vi "IIR Filter for N Chan.vi"(4 "optional IIR filter specifications":T3={"Lower PB"=100.0, "Upper PB"=0.0, "Lower SB"=200.0, "Upper SB"=0.0, "PB Gain"=0.0, "SB Gain"=-60.0, "Scale"=TRUE} {"PB Gain" format="%0.2f"; "SB Gain" format="%0.2f"; "Lower SB" format="%0.2p"; "Upper SB" format="%0.2f"; "Lower PB" format="%0.2p"; "Upper PB" format="%0.2f"}, 6 "IIR filter specifications":T4={"Topology"=enum."Butterworth", "Type"=enum."Lowpass", "Order"=1, "Lower Fc"=100.0, "Upper Fc"=200.0, "PB Ripple"=1.0, "SB Attenuation"=60.0} {"PB Ripple" format="%0.2f"; "SB Attenuation" format="%0.2f"; "Lower Fc" format="%0.2p"; "Upper Fc" format="%0.2p"}, 7 "reset filters":bool, 8 "error in (no error)":errorcluster, 10 "filter structure option":T1=10 items=["IIR 2nd Order"=0, "IIR 4th Order"=1, "Auto Select"=10], 11 "signal(s) in":waveform(dbl)[](array[waveform])) -> (0 "error out":errorcluster, 2 "filter information":T2 {"phase H(w)"."df" format="%.2p"; "phase H(w)"."f0" format="%.2p"; "phase H(w)"."Phase H(w)" format="%.2p"; "magnitude H(w)"."df" format="%.2p"; "magnitude H(w)"."f0" format="%.2p"; "magnitude H(w)"."Mag H(w)" format="%.2p"}, 3 "signal(s) out":waveform(dbl)[](array[waveform]))   [LabVIEW 2020, in "NI_MAPro.lvlib"]
doc: "Filters signals in either single or multiple waveforms. If you are filtering multiple waveforms, the VI maintains separate filter states for each waveform. The data types you wire to the <B>signal in</B> and <B>IIR filter specifications</B> inputs determine the polymorphic instance to use."
uses:
  NI_MAPro.lvlib
  Filter Structure Type.ctl
  NI_MABase.lvlib
  NI_AALBase.lvlib
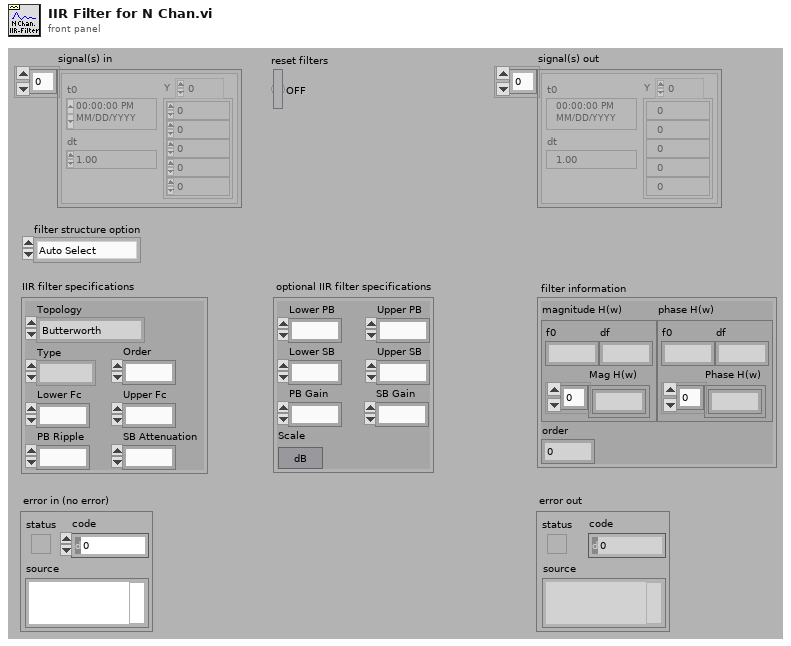
[diagram p1: front panel]
types:
  T1 = typedef "NI_AALBase.lvlib/Filter Structure Type.ctl" = u16
  T2 = cluster{"magnitude H(w)":cluster{"f0":dbl, "df":dbl, "Mag H(w)":dbl[]}, "phase H(w)":cluster{"f0":dbl, "df":dbl, "Phase H(w)":dbl[]}, "order":i32}
  T3 = cluster{"Lower PB":dbl, "Upper PB":dbl, "Lower SB":dbl, "Upper SB":dbl, "PB Gain":dbl, "SB Gain":dbl, "Scale":bool}
  T4 = cluster{"Topology":enum16{"Off", "Butterworth", "Chebyshev", "Inverse Chebyshev", "Elliptic", "Bessel"}, "Type":enum16{"Lowpass", "Highpass", "Bandpass", "Bandstop"}, "Order":i32, "Lower Fc":dbl, "Upper Fc":dbl, "PB Ripple":dbl, "SB Attenuation":dbl}
  T5 = cluster{"filter structure":enum32{"IIR 2nd Order", "IIR 4th Order"}, "Reverse Coefficients":dbl[], "Forward Coefficients":dbl[]}
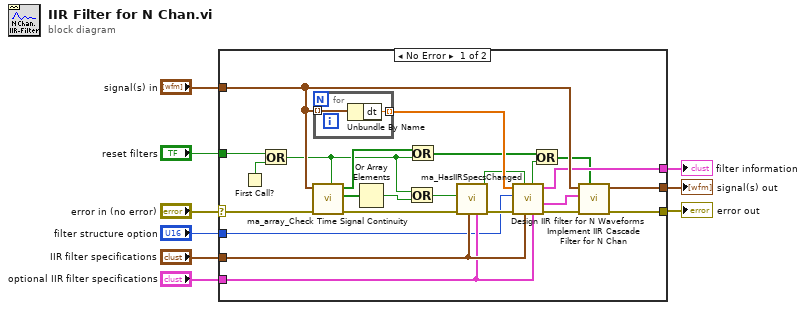
[diagram p0: block diagram]
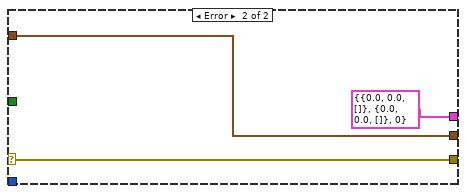
[diagram p2: hidden frame]
diagram:
  n1 = case shown="No Error" "error in (no error)" {
    selector: "error in (no error)" -> [w30 w37]
    tunnel: "signal(s) in" -> [w32 w38]
    tunnel: [w33 w37] -> w8
    tunnel: [w31 w38] -> w7
    tunnel: [w29 T2 {"magnitude H(w)"={"f0"=0.0, "df"=0.0, "Mag H(w)"=[]}, "phase H(w)"={"f0"=0.0, "df"=0.0, "Phase H(w)"=[]}, "order"=0} ("Filter Information")] -> w5
    tunnel: "reset filters" -> [w13 _]
    tunnel: "IIR filter specifications" -> [w12 _]
    tunnel: "optional IIR filter specifications" -> [w11 _]
    tunnel: "filter structure option" -> [w10 _]
    frame No Error {
      n2 = First Call?() -> (First Call?: T/F=w15:bool)
      n3 = Or(x=w13, y=w15) -> (x .or. y?=w14:bool)
      n4 = call "ma_array_Check Time Signal Continuity.vi"("Ignore input time stamp"=w14, "error in (no error)"=w30, "waveforms"=w32) -> ("error out"=w21:errorcluster, "dt changed"=w25:bool[], "t0 changed"=w17:bool[])  [unwired: 5 in, 1 out]
      n5 = for {
        tunnel: w32 -> [w35] mode=indexing
        tunnel: [w34] -> w26 mode=indexing
        n6 = Unbundle By Name(w35) -> ("dt"=w34:dbl)
      }
      n7 = Or Array Elements(Boolean array=w25) -> (logical OR=w18:bool)
      n8 = Or(x=w14, y=w18) -> (x .or. y?=w19:bool)
      n9 = Or(x=w17, y=w14) -> (x .or. y?=w16:bool[])
      n10 = call "ma_HasIIRSpecsChanged.vi"("optional IIR filter specifications"=w11, "IIR filter specifications"=w12, "error in (no error)"=w21, "redesign filter"=w19) -> ("error out"=w22:errorcluster, "ValsDifferent?"=w20:bool)  [unwired: 6 in]
      n11 = call "Design IIR filter for N Waveforms.vi"("Optional Filter Specifications"=w11, "Filter specifications"=w12, "Reset history"=w20, "error in"=w22, "filter structure option"=w10, "arrdt"=w26) -> ("error out"=w27:errorcluster, "IIR Filter Cluster"=w28:T5, "Filter Information"=w29:T2, "reset filters"=w24:bool)  [unwired: 2 in]
      n12 = Or(x=w16, y=w24) -> (x .or. y?=w23:bool[])
      n13 = call "Implement IIR Cascade Filter for N Chan.vi"("reset filter states"=w23, "error in (no error)"=w27, "IIR Filter Cluster"=w28, "arrWaveforms"=w32) -> ("error out"=w33:errorcluster, "arrFilteredWaveforms"=w31:waveform(dbl)[])  [unwired: 6 in]
    }
    frame Error {
    }
  }
  "error out" <- w8
  "signal(s) out" <- w7
  "filter information" <- w5
